vi "FTW-ERR-Replace.vi"(7 "Error Message":string, 9 "Error Code":i32, 11 "error in":errorcluster, 12 "Codes to Filter":i32[](array[numeric])) -> (15 "error out":errorcluster)   [LabVIEW 2015]
doc: "Overrides any incoming error that matches a code in the list with the new error"
panel:
  # "Inputs"
  # "Outputs"
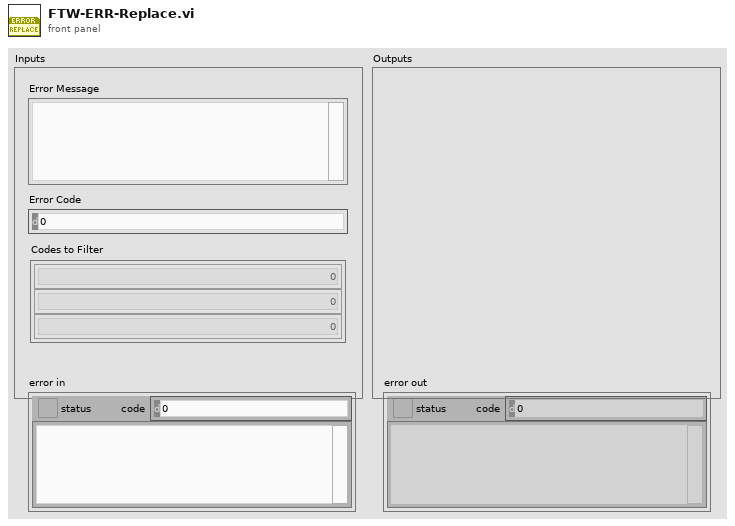
[diagram p1: front panel]
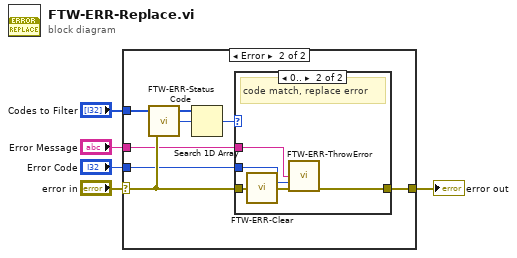
[diagram p0: block diagram]
diagram:
  n1 = case shown="Error" "error in" {
    selector: "error in" -> [w6 w12]
    tunnel: [w6 w13] -> w1
    tunnel: "Codes to Filter" -> [_ w10]
    tunnel: "Error Message" -> [_ w9]
    tunnel: "Error Code" -> [_ w8]
    frame No Error {
    }
    frame Error {
      n2 = call "FTW-ERR-StatusCode.vi"("error to check"=w12) -> ("Code"=w11:i32)
      n3 = Search 1D Array(1D array=w10, element=w11) -> (index of element=w7:i32)  [unwired: 1 in]
      n4 = case shown="0.." w7 {
        tunnel: [w14 w19] -> w13
        tunnel: w12 -> [w14 w18]
        tunnel: w9 -> [_ w17]
        tunnel: w8 -> [_ w16]
        frame ..-1 {
        }
        frame 0.. {
          # "code match, replace error"
          n5 = call "FTW-ERR-Clear.vi"("error to snuff"=w18) -> ("no error"=w15:errorcluster)
          n6 = call "FTW-ERR-ThrowError.vi"("Error Message"=w17, "Error Code"=w16, "error in"=w15) -> ("error out"=w19:errorcluster)  [unwired: 12 in]
        }
      }
    }
  }
  "error out" <- w1
